vi "ToscaTTL-Get Devices.vi"(11 "error in (no error)":errorcluster) -> (4 "Devices":refnum<class "TTLControlledDevice.lvclass">[](array[class]), 6 "Queues":refnum<queue>[](array[refnum]), 8 "Any devices?":bool, 15 "error out":errorcluster)   [LabVIEW 2020]
uses:
  Device Classes/Base Class/TTLControlledDevice.lvclass
  Control Classes/Base Class/TTLController.lvclass
  Sub VIs/Tosca-Globals.vi
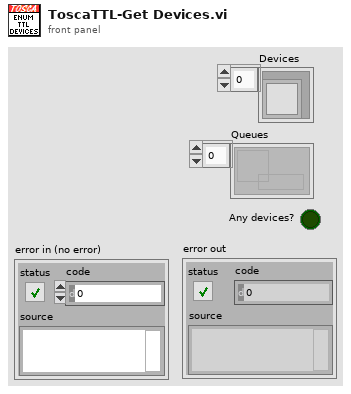
[diagram p1: front panel]
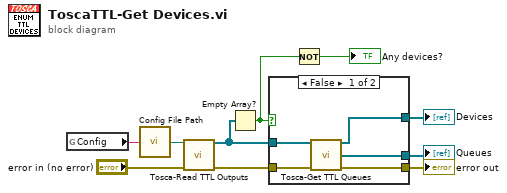
[diagram p0: block diagram]
diagram:
  n1 = global read "Tosca-Globals.vi" "Config"() -> (w7:string)
  n2 = call "Config File Path.vi"("AppName"=w7) -> ("Default config file name"=w6:path)
  n3 = call "Tosca-Read TTL Outputs.vi"("Connection File Path thru"=w6, "error in (no error)"="error in (no error)") -> ("Devices"=w3:refnum<class "TTLControlledDevice.lvclass">[], "error out"=w4:errorcluster)  [unwired: 12 in]
  n4 = Empty Array?(array=w3) -> (empty?=w2:bool)
  n5 = case shown="False" w2 {
    tunnel: w4 -> [w11 w17]
    tunnel: [w15 w16] -> w10
    tunnel: [w14 w17] -> w9
    tunnel: [w13 _] -> w8
    tunnel: w3 -> [w12 w16]
    frame False {
      n6 = call "Tosca-Get TTL Queues.vi"("Devices in"=w12, "error in (no error)"=w11) -> ("Devices out"=w15:refnum<class "TTLControlledDevice.lvclass">[], "Queues"=w13:refnum<queue>[], "error out"=w14:errorcluster)  [unwired: 11 in]
    }
    frame True {
    }
  }
  "Devices" <- w10
  "error out" <- w9
  "Queues" <- w8
  n7 = Not(x=w2) -> (.not. x?=→"Any devices?":bool)
